vi "Add XY (single).vi"(8 "error in (no error)":errorcluster, 9 "y":cluster{"X-array":dbl[], "Y-array":dbl[]}, 10 "x":cluster{"X-array":dbl[], "Y-array":dbl[]}, 11 "XY-data":cluster{"X-array":dbl[], "Y-array":dbl[]}) -> (0 "error out":errorcluster, 3 "XY-data out":cluster{"X-array":dbl[], "Y-array":dbl[]} {"Y-array" format="%.2p"; "X-array" format="%.2p"})   [LabVIEW 2019, in "xy_utilities.lvlib"]
doc: "Add <b>x</b>'s x array to the x array of <b>XY-data</b>\nAdd <b>y</b>'s y array to the y array of <b>XY-data</b>\n\nWire data to the data input to determine the polymorphic instance to use or manually select the instance."
uses:
  xy_utilities.lvlib
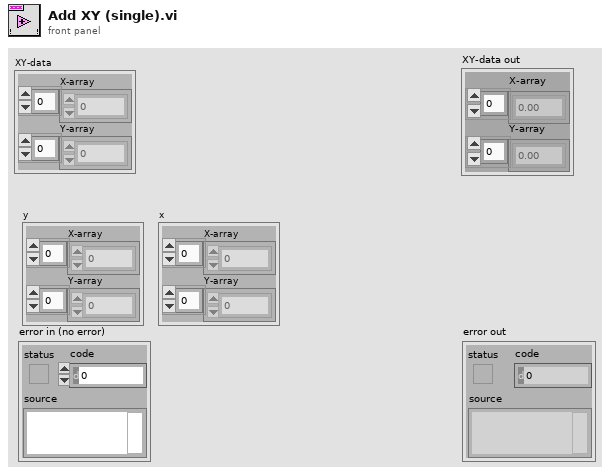
[diagram p1: front panel]
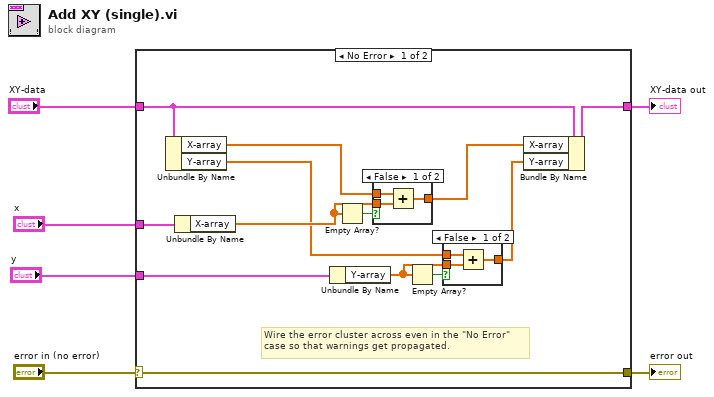
[diagram p0: block diagram]
diagram:
  n1 = case shown="No Error" "error in (no error)" {
    selector: "error in (no error)" -> [w19 w29]
    tunnel: [w19 w29] -> w5
    tunnel: "XY-data" -> [w18 w28]
    tunnel: [w17 w28] -> w3
    tunnel: "y" -> [w16 _]
    tunnel: "x" -> [w15 _]
    frame No Error {
      # "Wire the error cluster across even in the \"No Error\"\ncase so that warnings get propagated."
      n2 = Unbundle By Name(w18) -> ("X-array"=w10:dbl[], "Y-array"=w8:dbl[])
      n3 = Unbundle By Name(w15) -> ("X-array"=w9:dbl[])
      n4 = Unbundle By Name(w16) -> ("Y-array"=w11:dbl[])
      n5 = Empty Array?(array=w9) -> (empty?=w13:bool)
      n6 = case shown="False" w13 {
        tunnel: w9 -> [w26 _]
        tunnel: w10 -> [w25 w27]
        tunnel: [w24 w27] -> w14
        frame False {
          n7 = Add(x=w25, y=w26) -> (x+y=w24:dbl[])
        }
        frame True {
        }
      }
      n8 = Empty Array?(array=w11) -> (empty?=w12:bool)
      n9 = case shown="False" w12 {
        tunnel: w11 -> [w22 _]
        tunnel: w8 -> [w21 w23]
        tunnel: [w20 w23] -> w7
        frame False {
          n10 = Add(x=w21, y=w22) -> (x+y=w20:dbl[])
        }
        frame True {
        }
      }
      n11 = Bundle By Name(cluster=w18, "X-array"=w14, "Y-array"=w7) -> (w17:cluster{"X-array":dbl[], "Y-array":dbl[]})
    }
    frame Error {
    }
  }
  "error out" <- w5
  "XY-data out" <- w3
